vi "Analogue 0 (Angle, Optical Switch).vi"(11 "Port Number":u32(knob) scale=0.0..3.0) -> (0 "pin 6":fxp<+/-,20,5> format="%.2g", 1 "pin 5":fxp<+/-,20,5> format="%.2g", 2 "pin 4":fxp<+/-,20,5> format="%.2g", 3 "pin 3":fxp<+/-,20,5> format="%.2g", 8 "pin 2":fxp<+/-,20,5> format="%.2g", 9 "pin 1":fxp<+/-,20,5> format="%.2g")   [LabVIEW 2023]
uses:
  <vilib>/rvi/eio/common/nirviEmuTemplateMethod_errors.vi
  <vilib>/eio/EIONode/EIONode.xnode
panel:
  # "Analogue 0: Optical Switch, Angle"
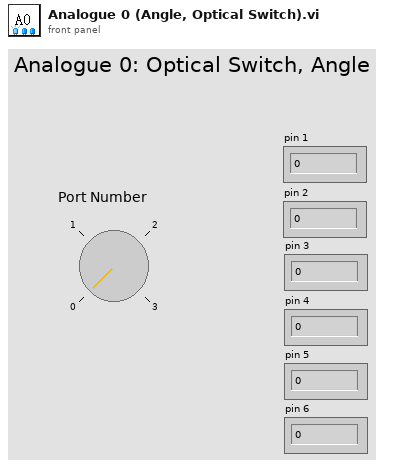
[diagram p1: front panel]
types:
  T1 = cluster{"pin 3":sgl, "pin 5":sgl, "pin 6":sgl, "pin 2":sgl, "pin 4":sgl, "pin 1":fxp<+/-,20,5>}[]
  T2 = cluster{"pin 1":fxp<+/-,20,5>, "pin 2":fxp<+/-,20,5>, "pin 3":fxp<+/-,20,5>, "pin 4":fxp<+/-,20,5>, "pin 5":fxp<+/-,20,5>, "pin 6":fxp<+/-,20,5>}[]
  T3 = cluster{"pin 1":fxp<+/-,20,5>, "pin 2":fxp<+/-,20,5>, "pin 3":fxp<+/-,20,5>, "pin 4":fxp<+/-,20,5>, "pin 5":fxp<+/-,20,5>, "pin 6":fxp<+/-,20,5>}
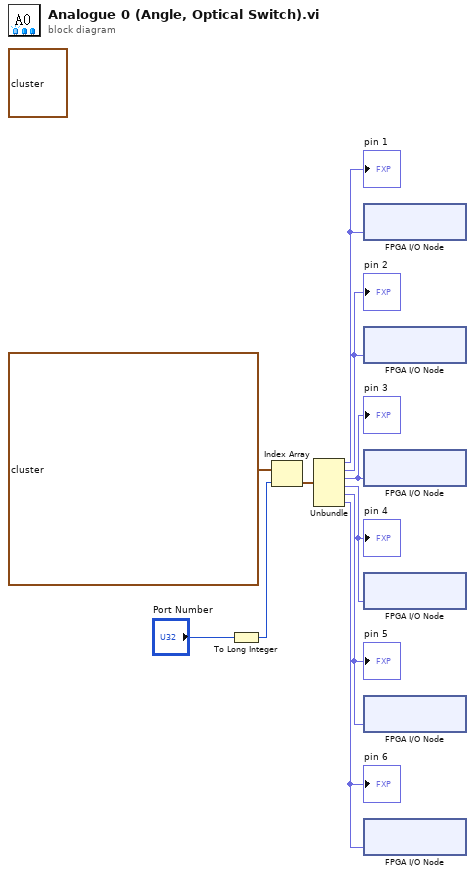
[diagram p0: block diagram]
diagram:
  (unwired) T1 [{"pin 3"=0.0, "pin 5"=0.0, "pin 6"=0.0, "pin 2"=4.5, "pin 4"=4.5, "pin 1"=0.0}, {"pin 3"=4.5, "pin 5"=0.0, "pin 6"=0.0, "pin 2"=4.5, "pin 4"=0.0, "pin 1"=0.0}, {"pin 3"=0.0, "pin 5"=0.0, "pin 6"=4.5, "pin 2"=0.0, "pin 4"=0.0, "pin 1"=0.0}, {"pin 3"=0.0, "pin 5"=4.5, "pin 6"=0.0, "pin 2"=0.0, "pin 4"=0.0, "pin 1"=0.0}]
  n1 = To Long Integer(number="Port Number") -> (32bit integer=w1:i32)
  n2 = Index Array(array=T2 [{"pin 1"=0.0, "pin 2"=4.5, "pin 3"=0.0, "pin 4"=4.5, "pin 5"=0.0, "pin 6"=0.0}, {"pin 1"=0.0, "pin 2"=4.5, "pin 3"=4.5, "pin 4"=0.0, "pin 5"=0.0, "pin 6"=0.0}, {"pin 1"=4.5, "pin 2"=0.0, "pin 3"=0.0, "pin 4"=0.0, "pin 5"=0.0, "pin 6"=4.5}, {"pin 1"=4.5, "pin 2"=0.0, "pin 3"=0.0, "pin 4"=0.0, "pin 5"=4.5, "pin 6"=0.0}], index=w1) -> (element=w9:T3)
  n3 = Unbundle(w9) -> ("pin 1"=w8:fxp<+/-,20,5>, "pin 2"=w7:fxp<+/-,20,5>, "pin 3"=w6:fxp<+/-,20,5>, "pin 4"=w5:fxp<+/-,20,5>, "pin 5"=w4:fxp<+/-,20,5>, "pin 6"=w3:fxp<+/-,20,5>)
  "pin 1" <- w8
  "pin 2" <- w7
  "pin 3" <- w6
  "pin 4" <- w5
  "pin 5" <- w4
  "pin 6" <- w3
  n4 = xnode "FPGA I/O Node"("Mod3/AO0"=w8) -> ()  [unwired: 1 in, 1 out]
  n5 = xnode "FPGA I/O Node"("Mod3/AO1"=w7) -> ()  [unwired: 1 in, 1 out]
  n6 = xnode "FPGA I/O Node"("Mod3/AO2"=w6) -> ()  [unwired: 1 in, 1 out]
  n7 = xnode "FPGA I/O Node"("Mod3/AO3"=w5) -> ()  [unwired: 1 in, 1 out]
  n8 = xnode "FPGA I/O Node"("Mod3/AO4"=w4) -> ()  [unwired: 1 in, 1 out]
  n9 = xnode "FPGA I/O Node"("Mod3/AO5"=w3) -> ()  [unwired: 1 in, 1 out]
